vi "Initialize Streaming Data.vi"(8 "error in (no error)":errorcluster, 11 "Device Ref in":T7=18446744073709551615 format="%.0x") -> (0 "error out":errorcluster, 1 "Group Sample Spec":T1 {"Decimation Ref" format="%.0x"; "Block Refs"."Data Reference" format="%.0x"}, 2 "Streaming spec":T4, 3 "Device Ref out":T7=18446744073709551615 format="%.0x", 4 "Group Size":i32, 5 "FIFO % Ref":T3 format="%.0x")   [LabVIEW 2024, in "Nominal Client Engine.lvlib"]
uses:
  Nominal Client Engine.lvlib
  <vilib>/NI VeriStand/Custom Device API/Custom Device Item Ref.ctl
  <vilib>/NI VeriStand/Custom Device API/Data Reference.ctl
  Streaming Specification.ctl
  Group Buffer Data.ctl
  Property Specification.ctl
  Group Sample Specification.ctl
  <vilib>/NI VeriStand/Custom Device API/Block Data Reference.ctl
  <vilib>/NI VeriStand/Custom Device API/Data Access Type.ctl
  <vilib>/NI VeriStand/Custom Device API/Custom Device API.lvlib
  <vilib>/NI VeriStand/Custom Device Tools/Custom Device Utility Library/Custom Device Utility Library.lvlib
  <vilib>/NI VeriStand/Custom Device Tools/Custom Device Utility Library/NI VeriStand - Search for Item by Property.vi
  Scripting/Nominal Client Scripting.lvlib
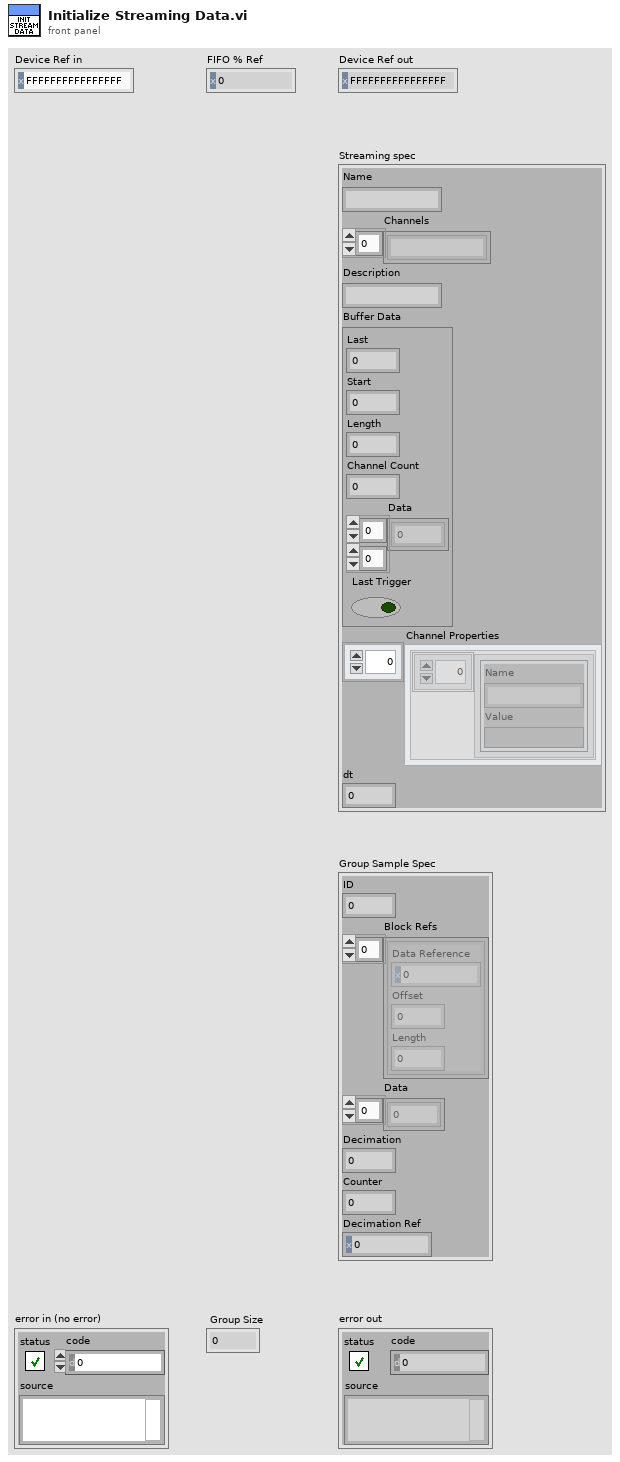
[diagram p1: front panel]
types:
  T1 = typedef "Nominal Client Engine.lvlib/Group Sample Specification.ctl" = cluster{"ID":dbl, "Block Refs":T2[], "Data":dbl[], "Decimation":i32, "Counter":i32, "Decimation Ref":T3}
  T2 = typedef "Custom Device API.lvlib/Block Data Reference.ctl" = cluster{"Data Reference":T3, "Offset":u64, "Length":u64}
  T3 = typedef "Custom Device API.lvlib/Data Reference.ctl" = i32
  T4 = typedef "Nominal Client Engine.lvlib/Streaming Specification.ctl" = cluster{"Name":string, "Channels":string[], "Description":string, "Buffer Data":T5, "Channel Properties":cluster{"Array":T6[]}[], "dt":dbl}
  T5 = typedef "Nominal Client Engine.lvlib/Group Buffer Data.ctl" = cluster{"Last":i32, "Start":i32, "Length":i32, "Channel Count":i32, "Data":dbl[][], "Last Trigger":bool}
  T6 = typedef "Nominal Client Engine.lvlib/Property Specification.ctl" = cluster{"Name":string, "Value":variant}
  T7 = typedef "Custom Device API.lvlib/Custom Device Item Ref.ctl" = u64
  T8 = typedef "Custom Device API.lvlib/Data Access Type.ctl" = enum16{"Read", "Write"}
  T9 = typedef "Custom Device API.lvlib/Custom Device Item Info.ctl" = cluster{"Name":string, "Is Channel":bool, "GUID":string, "Is Waveform":bool}
  T10 = cluster{cluster{"Name":string, "Variant":variant}[]}
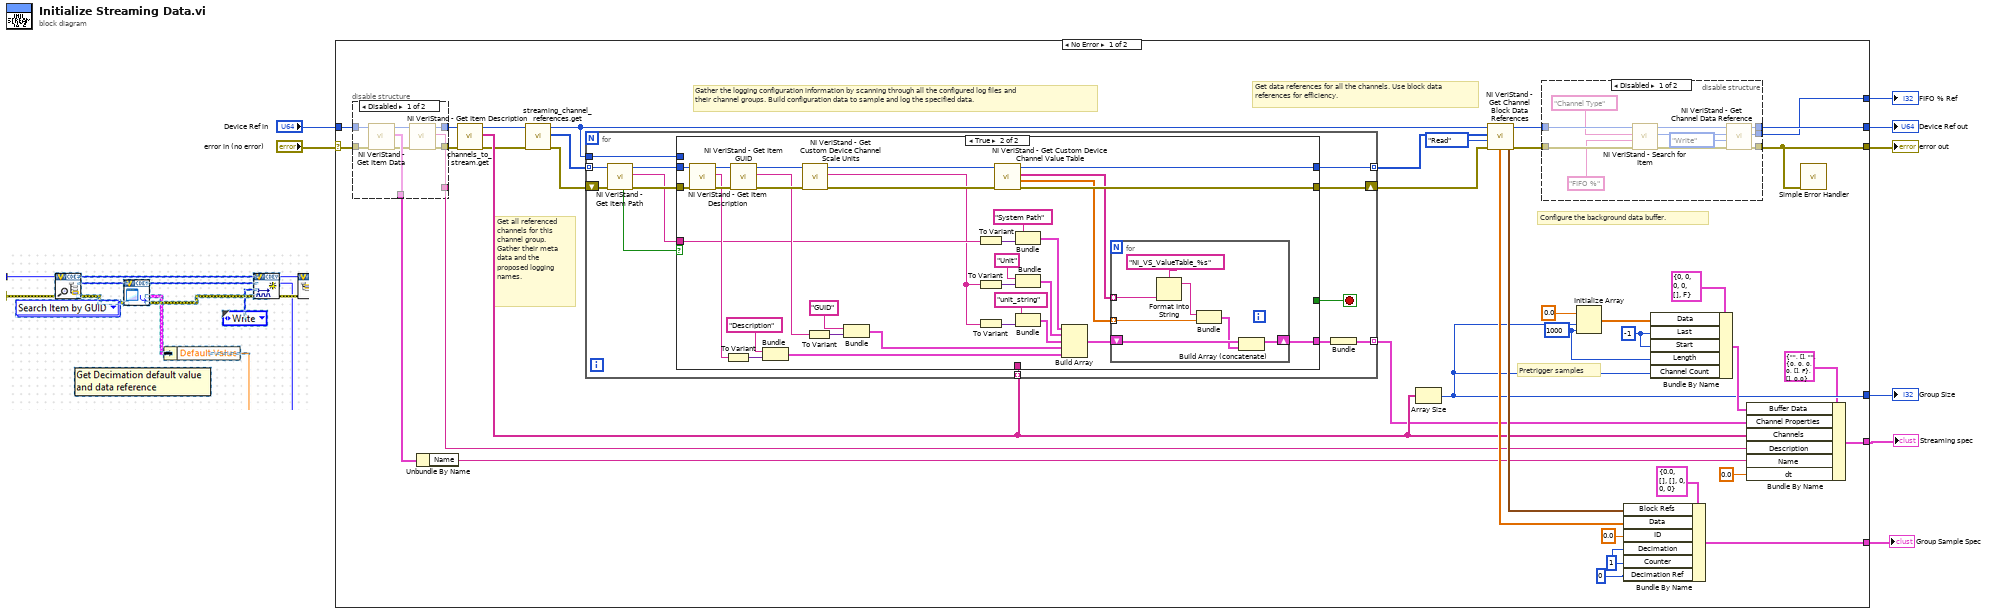
[diagram p0: block diagram]
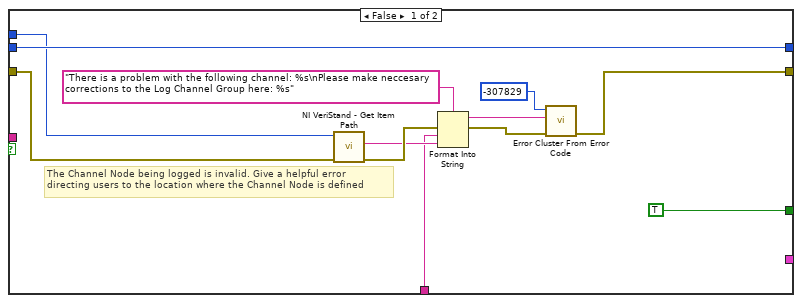
[diagram p4: hidden frame]
diagram:
  n1 = case shown="No Error" "error in (no error)" {
    selector: "error in (no error)" -> [w13 w137]
    tunnel: [w9 w137] -> w8
    tunnel: "Device Ref in" -> [w14 w136]
    tunnel: [w45 w136] -> w5
    tunnel: [w20 _] -> w4
    tunnel: [w44 _] -> w3
    tunnel: [w23 _] -> w1
    tunnel: [w21 _] -> w2
    frame No Error {
      w19 = 1000 ("dimension size")
      w35 = -1 ("Last")
      w10 = 1 ("Counter")
      # "Pretrigger samples"
      # "Get data references for all the channels. Use block data references for efficiency."
      # "Configure the background data buffer."
      # "Get all referenced channels for this channel group. Gather their meta data and the proposed logging names."
      # "Gather the logging configuration information by scanning through all the configured log files and their channel groups. Build configuration data to sample and log the specified data."
      n2 = disable-structure shown="Disabled" {
        disable-tunnel: [w68 _] -> w42
        disable-tunnel: [w66 _] -> w37
        disable-tunnel: [w65 w70] -> w30
        disable-tunnel: [w64 w69] -> w29
        disable-tunnel: w14 -> [w62 w70]
        disable-tunnel: w13 -> [w61 w69]
        frame Disabled {
          n3 = call <vilib>:"NI VeriStand - Get Item Data.vi"("error in (no error)"=w61, "Item Ref in"=w62) -> ("error out"=w67:errorcluster, "Item Info"=w68:T9, "Item Ref out"=w63:T7)  [unwired: 7 out]
          n4 = call <vilib>:"NI VeriStand - Get Item Description.vi"("error in (no error)"=w67, "Item Ref in"=w63) -> ("error out"=w64:errorcluster, "Description"=w66:string, "Item Ref out"=w65:T7)  [unwired: 7 out]
        }
        frame Enabled {
        }
      }
      n5 = Unbundle By Name(w42) -> ("Name"=w32:string)
      n6 = call "channels_to_stream.get.vi"("error in (no error)"=w29, "Nominal IO Client in"=w30) -> ("error out"=w26:errorcluster, "Channels to Stream"=w31:string[], "Nominal IO Client out"=w28:T7)  [unwired: 6 in, 1 out]
      n7 = call "streaming_channel_references.get.vi"("error in (no error)"=w26, "Item Ref in"=w28) -> ("error out"=w27:errorcluster, "Streaming Channel Refs"=w25:T7[], "Item Ref out"=w24:T7)  [unwired: 7 in]
      n8 = for {
        shift-right: [w75] -> w39
        shift-left: w27 -> [w80]
        tunnel: [w76] -> w41 mode=indexing
        tunnel: [w82] -> w16 mode=indexing
        tunnel: w25 -> [w81] mode=indexing
        tunnel: w24 -> [w73]
        tunnel: w31 -> [w72] mode=indexing
        stop <- w71 stop-if-true
        n9 = call <vilib>:"NI VeriStand - Get Item Path.vi"("error in (no error)"=w80, "Item Ref in"=w81) -> ("error out"=w79:errorcluster, "Path"=w77:string, "Item Ref out"=w78:T7, "Found"=w74:bool)  [unwired: 6 in]
        n10 = case shown="True" w74 {
          tunnel: [_ w99] -> w83
          tunnel: w79 -> [w93 w110]
          tunnel: w78 -> [w95 w109]
          tunnel: w77 -> [_ w104]
          tunnel: [w95 w101] -> w76
          tunnel: [w87 w100] -> w75
          tunnel: w73 -> [w94 _]
          tunnel: w72 -> [w85 _]
          tunnel: [TRUE _] -> w71
          frame False {
            # "The Channel Node being logged is invalid. Give a helpful error \ndirecting users to the location where the Channel Node is defined"
            n11 = call <vilib>:"NI VeriStand - Get Item Path.vi"("error in (no error)"=w93, "Item Ref in"=w94) -> ("error out"=w88:errorcluster, "Path"=w86:string)  [unwired: 6 in, 2 out]
            n12 = Format Into String(format string="There is a problem with the following channel: %s\nPlease make neccesary corrections to the Log Channel Group here: %s" ("initial string"), error in=w88, w85, w86) -> (resulting string=w91:string, error out=w89:errorcluster)  [unwired: 1 in]
            n13 = call <vilib>:"Error Cluster From Error Code.vi"("error in (no error)"=w89, "error message (\"\")"=w91, "error code (0)"=-307829 ("Code")) -> ("error out"=w87:errorcluster)  [unwired: 6 in]
          }
          frame True {
            n14 = call <vilib>:"NI VeriStand - Get Item Description.vi"("error in (no error)"=w110, "Item Ref in"=w109) -> ("error out"=w125:errorcluster, "Description"=w124:string, "Item Ref out"=w126:T7)  [unwired: 7 out]
            n15 = To Variant(anything=w124) -> (Variant=w123:variant)
            n16 = call <vilib>:"NI VeriStand - Get Item GUID.vi"("error in (no error)"=w125, "Item Ref in"=w126) -> ("error out"=w127:errorcluster, "GUID"=w119:string, "Item Ref out"=w105:T7)  [unwired: 7 out]
            n17 = Bundle("Name"="Description", "Variant"=w123) -> (w117:cluster{"Name":string, "Variant":variant})  [unwired: 1 out]
            n18 = call <vilib>:"NI VeriStand - Get Custom Device Channel Scale Units.vi"("error in (no error)"=w127, "Channel Ref in"=w105) -> ("error out"=w128:errorcluster, "ScaleUnits"=w103:string, "Channel Ref out"=w102:T7)  [unwired: 7 in]
            n19 = To Variant(anything=w119) -> (Variant=w120:variant)
            n20 = Bundle("Name"="GUID", "Variant"=w120) -> (w118:cluster{"Name":string, "Variant":variant})  [unwired: 1 out]
            n21 = To Variant(anything=w104) -> (Variant=w112:variant)
            n22 = To Variant(anything=w103) -> (Variant=w116:variant)
            n23 = To Variant(anything=w103) -> (Variant=w107:variant)
            n24 = call <vilib>:"NI VeriStand - Get Custom Device Channel Value Table.vi"("error in (no error)"=w128, "Channel Ref in"=w102) -> ("error out"=w100:errorcluster, "Values"=w96:dbl[], "Names"=w97:string[], "Channel Ref out"=w101:T7)  [unwired: 6 in]
            n25 = Bundle("Name"="System Path", "Variant"=w112) -> (w111:cluster{"Name":string, "Variant":variant})  [unwired: 1 out]
            n26 = Bundle("Name"="Unit", "Variant"=w116) -> (w114:cluster{"Name":string, "Variant":variant})  [unwired: 1 out]
            n27 = Bundle("Name"="unit_string", "Variant"=w107) -> (w106:cluster{"Name":string, "Variant":variant})  [unwired: 1 out]
            n28 = Build Array(w111, w114, w106, w118, w117) -> (w98:cluster{"Name":string, "Variant":variant}[])
            n29 = for {
              shift-right: [w134] -> w99
              shift-left: w98 -> [w135]
              tunnel: w97 -> [w131] mode=indexing
              tunnel: w96 -> [w130] mode=indexing
              n30 = Format Into String(format string="NI_VS_ValueTable_%s" ("Name"), w131) -> (resulting string=w132:string)  [unwired: 2 in, 1 out]
              n31 = Bundle(w132, w130) -> (w129:cluster{string, dbl})  [unwired: 1 out]
              n32 = Build Array (concatenate)(w135, w129) -> (w134:cluster{"Name":string, "Variant":variant}[])
            }
          }
        }
        n33 = Bundle(w83) -> (w82:T10)  [unwired: 1 in]
      }
      n34 = Array Size(array=w31) -> (size(s)=w20:i32)
      n35 = call <vilib>:"NI VeriStand - Get Channel Block Data References.vi"("error in (no error)"=w39, "Access"=Data_Access_Type."Read", "Channel Refs"=w41, "Device Ref in"=w24) -> ("error out"=w46:errorcluster, "Values Array"=w43:dbl[], "Block Data Refs"=w38:T2[], "Device Ref out"=w47:T7)  [unwired: 4 out]
      n36 = disable-structure shown="Disabled" {
        disable-tunnel: w47 -> [w58 w60]
        disable-tunnel: w46 -> [w57 w59]
        disable-tunnel: [w56 w60] -> w45
        disable-tunnel: [w55 _] -> w44
        disable-tunnel: [w48 w59] -> w9
        frame Disabled {
          n37 = call-poly <vilib>:"NI VeriStand - Search for Item.vi"("error in"=w57, "Property Value"="FIFO %" ("String"), "Property Name"="Channel Type" ("String"), "Section Ref in"=w58) -> ("error out"=w50:errorcluster, "Item Ref"=w51:T7, "Section Ref out"=w52:T7)  [unwired: 4 in, 1 out]
          n38 = call <vilib>:"NI VeriStand - Get Channel Data Reference.vi"("error in (no error)"=w50, "Access"=Data_Access_Type."Write", "Channel Ref in"=w51, "Device Ref in"=w52) -> ("error out"=w48:errorcluster, "Channel Data Reference"=w55:T3, "Device Ref out"=w56:T7)  [unwired: 5 in]
        }
        frame Enabled {
        }
      }
      n39 = Initialize Array(0.0 ("element"), w20, w19) -> (w33:dbl[][])
      n40 = Bundle By Name(cluster=T1 {"ID"=0.0, "Block Refs"=[], "Data"=[], "Decimation"=0, "Counter"=0, "Decimation Ref"=0} ("Group Sample Spec"), "Block Refs"=w38, "Data"=w43, "ID"=0.0, "Decimation"=w10, "Counter"=w10, "Decimation Ref"=T3 0) -> (w23:T1)
      n41 = Bundle By Name(cluster=T5 {"Last"=0, "Start"=0, "Length"=0, "Channel Count"=0, "Data"=[], "Last Trigger"=FALSE} ("Buffer Data"), "Data"=w33, "Last"=w35, "Start"=w35, "Length"=w19, "Channel Count"=w20) -> (w36:T5)
      n42 = Bundle By Name(cluster=T4 {"Name"="", "Channels"=[], "Description"="", "Buffer Data"={"Last"=0, "Start"=0, "Length"=0, "Channel Count"=0, "Data"=[], "Last Trigger"=FALSE}, "Channel Properties"=[], "dt"=0.0} ("Streaming spec"), "Buffer Data"=w36, "Channel Properties"=w16, "Channels"=w31, "Description"=w37, "Name"=w32, "dt"=0.0) -> (w21:T4)
      n43 = call <vilib>:"Simple Error Handler.vi"("error in (no error)"=w9) -> ()  [unwired: 4 in, 5 out]
    }
    frame Error {
    }
  }
  "error out" <- w8
  "Device Ref out" <- w5
  "Group Size" <- w4
  "FIFO % Ref" <- w3
  "Streaming spec" <- w2
  "Group Sample Spec" <- w1
